vi "BlendSuggestionsToGoStraight.vi"(9 "LuffToSailSuggestion":dbl, 10 "BalanceRudderSailSuggestion":dbl, 11 "WindToSailLookup":dbl) -> (3 "BlendedSailSuggestion":dbl)   [LabVIEW 2012]
doc: "This VI takes in suggestions for\n1) Simple sail lookup by Point of Sail\n2) How to move the sails to balance the rudder\n3) How to move the sails to stop luffing\n\nThis VI is intended to generally pass through #1 unimpeded, but gradually filter in the advice from #2 and #3 over time. The mechanism for this will be either increasing the gain of suggestions (2, 3) as the boat nears 'cruising' velocity or indcreasing the gain as a function of the time spent in the 'go straight' boat state."
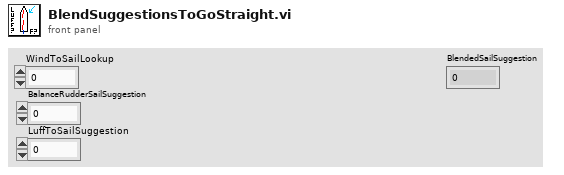
[diagram p1: front panel]
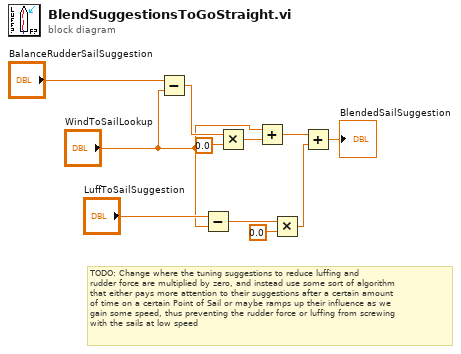
[diagram p0: block diagram]
diagram:
  # "TODO: Change where the tuning suggestions to reduce luffing and\nrudder force are multiplied by zero, and instead use some sort of algorithm\nthat either pays more attention to their suggestions after a certain amount\nof time on a certain Point of Sail or maybe ramps up their influence as we\ngain some speed, thus preventing the rudder force or luffing from screwing\nwith the sails at low speed"
  n1 = Subtract(x="BalanceRudderSailSuggestion", y="WindToSailLookup") -> (x-y=w8:dbl)
  n2 = Subtract(x="LuffToSailSuggestion", y="WindToSailLookup") -> (x-y=w5:dbl)
  n3 = Multiply(x=w8, y=0.0) -> (x*y=w2:dbl)
  n4 = Add(x="WindToSailLookup", y=w2) -> (x+y=w11:dbl)
  n5 = Multiply(x=w5, y=0.0) -> (x*y=w1:dbl)
  n6 = Add(x=w11, y=w1) -> (x+y=→"BlendedSailSuggestion":dbl)
